vi "CRC16.vi"() -> ()   [LabVIEW 2011]
panel:
  out "Hi":u8 format="%x"
  out "Lo":u8 format="%x"
  in  "数组":u8[](array[numeric])
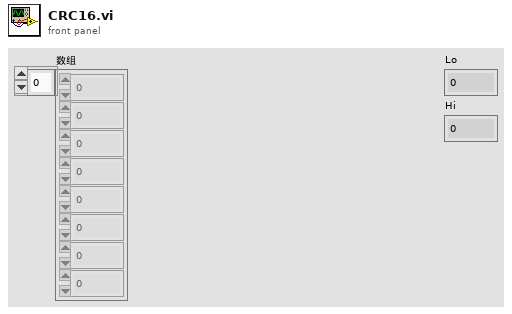
[diagram p1: front panel]
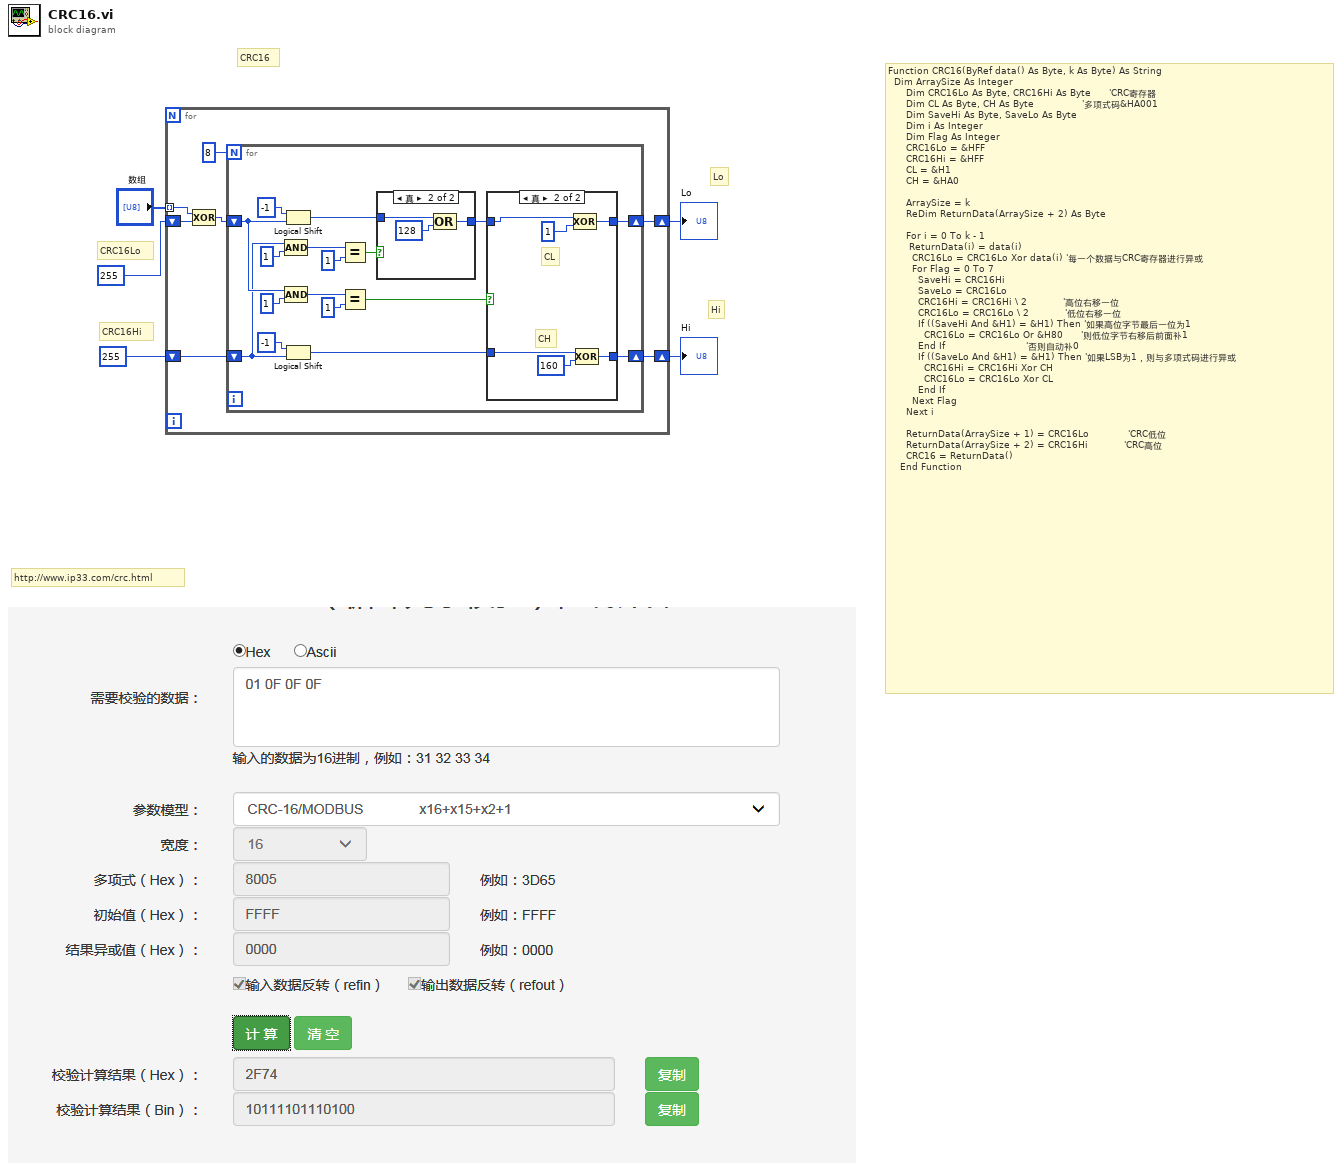
[diagram p0: block diagram]
diagram:
  # "Function CRC16(ByRef data() As Byte, k As Byte) As String\n  Dim ArraySize As Integer\n      Dim CRC16Lo As Byte, CRC16Hi As Byte      'CRC寄存器\n      Dim CL As Byte, CH As Byte                '多项式码&HA001\n      Dim SaveHi As Byte, SaveLo As Byte\n      Dim i As Integer\n      Dim Flag As Integer\n      CRC16Lo = &HFF\n      CRC16Hi = &HFF\n      CL = &H1\n      CH = &HA0\n      \n      ArraySize = k\n      ReDim ReturnData(ArraySize + 2) As Byte\n     \n      For i = 0 To k - 1\n       ReturnData(i) = data(i)\n        CRC16Lo = CRC16Lo Xor data(i) '每一个数据与CRC寄存器进行异或\n        For Flag = 0 To 7\n          SaveHi = CRC16Hi\n          SaveLo = CRC16Lo\n          CRC16Hi = CRC16Hi \\ 2            '高位右移一位\n          CRC16Lo = CRC16Lo \\ 2            '低位右移一位\n          If ((SaveHi And &H1) = &H1) Then '如果高位字节最后一位为1\n            CRC16Lo = CRC16Lo Or &H80      '则低位字节右移后前面补1\n          End If                           '否则自动补0\n          If ((SaveLo And &H1) = &H1) Then '如果LSB为1，则与多项式码进行异或\n            CRC16Hi = CRC16Hi Xor CH\n            CRC16Lo = CRC16Lo Xor CL\n          End If\n        Next Flag\n      Next i\n      \n      ReturnData(ArraySize + 1) = CRC16Lo             'CRC低位\n      ReturnData(ArraySize + 2) = CRC16Hi            'CRC高位\n      CRC16 = ReturnData()\n    End Function"
  # "http://www.ip33.com/crc.html"
  # "CRC16"
  # "Lo"
  # "Hi"
  # "CRC16Hi"
  # "CRC16Lo"
  n1 = for {
    tunnel: "数组" -> [w12] mode=indexing
    shift-right: [w7] -> w2
    shift-left: u8 255 ("值") -> [w11]
    shift-right: [w6] -> w1
    shift-left: u8 255 ("值") -> [w8]
    n2 = Compound Arithmetic op=XOR(w12, w11) -> (w9:u8)
    n3 = for {
      N: 8 -> [_]
      shift-right: [w14] -> w7
      shift-left: w9 -> [w20]
      shift-right: [w13] -> w6
      shift-left: w8 -> [w17]
      n4 = Logical Shift(y=i8 -1, x=w20) -> (x << y=w18:u8)
      n5 = Logical Shift(y=i8 -1, x=w17) -> (x << y=w15:u8)
      n6 = Compound Arithmetic op=AND(w17, u8 1 ("值")) -> (w25:u8)
      n7 = Compound Arithmetic op=AND(w20, u8 1 ("值")) -> (w28:u8)
      n8 = Equal?(x=w25, y=u8 1) -> (x = y?=w22:bool)
      n9 = Equal?(x=w28, y=u8 1) -> (x = y?=w23:bool)
      n10 = case shown="真" w22 {
        tunnel: w18 -> [w30 w33]
        tunnel: [w30 w31] -> w21
        frame False {
        }
        frame True {
          n11 = Compound Arithmetic op=OR(w33, u8 128 ("值")) -> (w31:u8)
        }
      }
      n12 = case shown="真" w23 {
        tunnel: w21 -> [w34 w41]
        tunnel: w15 -> [w35 w39]
        tunnel: [w35 w37] -> w13
        tunnel: [w34 w36] -> w14
        frame False {
        }
        frame True {
          # "CH"
          # "CL"
          n13 = Compound Arithmetic op=XOR(w41, u8 1 ("值")) -> (w36:u8)
          n14 = Compound Arithmetic op=XOR(w39, u8 160 ("值")) -> (w37:u8)
        }
      }
    }
  }
  "Lo" <- w2
  "Hi" <- w1
